vi "NI Selection.vi"(7 "error in (no error)":errorcluster) -> (0 "NI 2":tag, 1 "NI 1":tag, 2 "Ok/Cancel":enum16{"Ok", "Cancel"}(ring), 3 "error out":errorcluster)   [LabVIEW 2017]
uses:
  <resource>/objmgr/daqmx.rc
panel:
  in  "NI2":tag
  in  "NI1":tag
  in  "Cancel Button":bool
  in  "OK Button":bool
  # "PLease Choose Correct NI Serial Number"
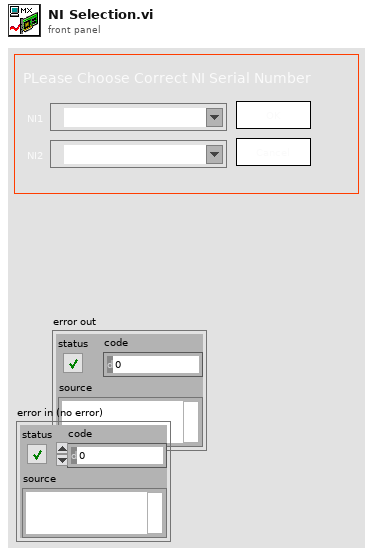
[diagram p1: front panel]
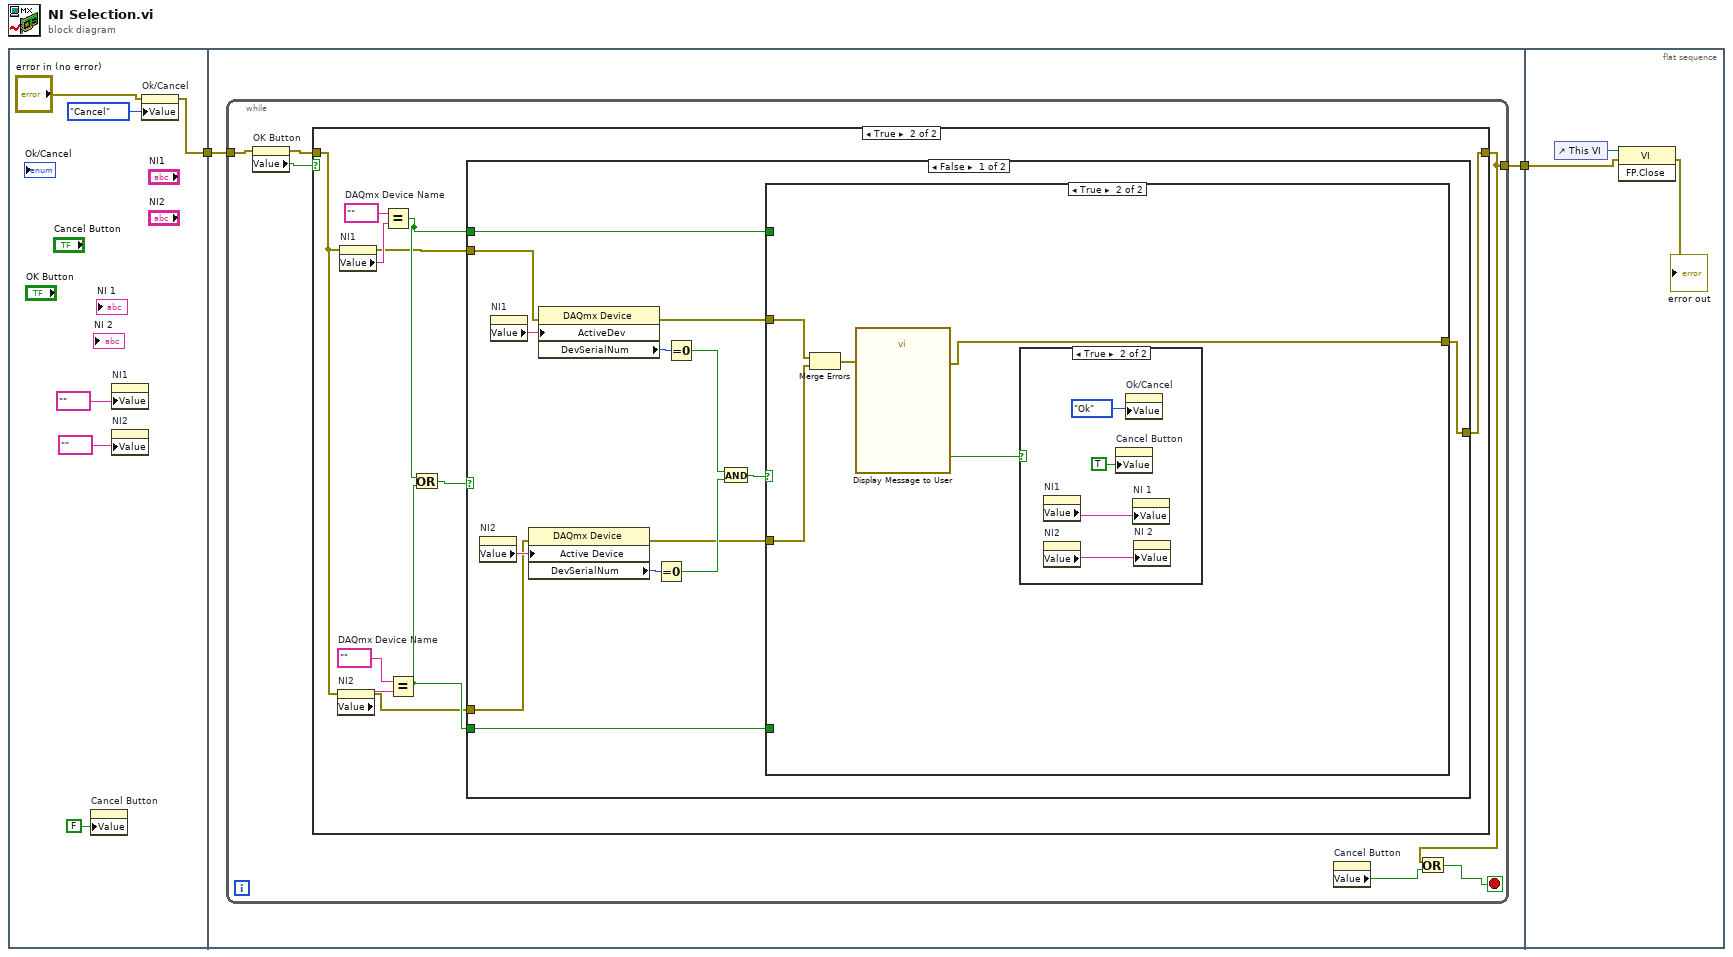
[diagram p0: block diagram]
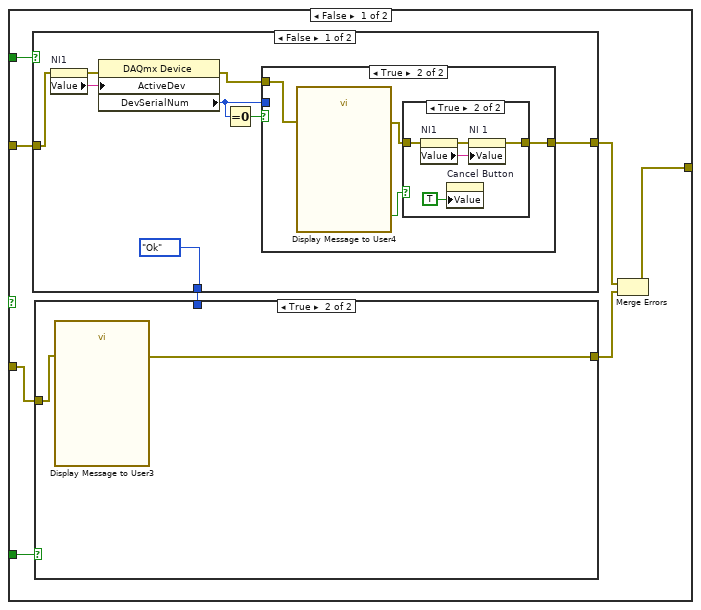
[diagram p3: hidden frame]
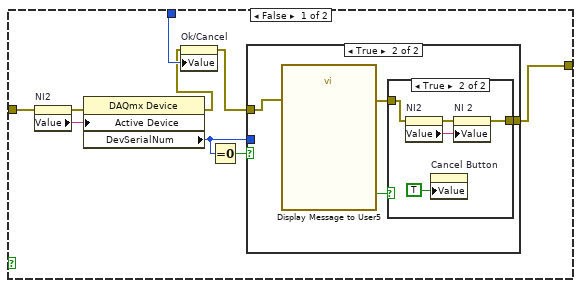
[diagram p4: hidden frame]
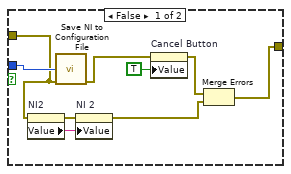
[diagram p5: hidden frame]
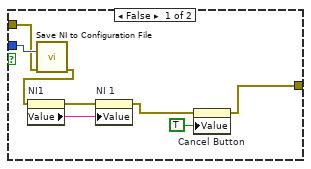
[diagram p7: hidden frame]
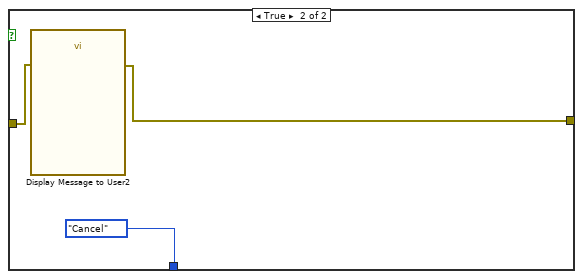
[diagram p9: hidden frame]
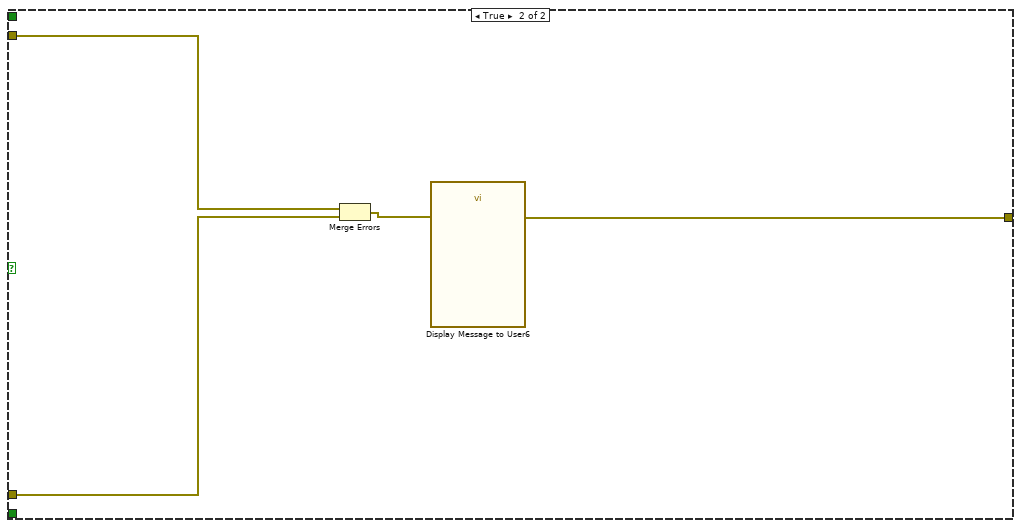
[diagram p11: hidden frame]
diagram:
  n1 = flat-sequence {
    tunnel: [w4] -> w2
    tunnel: w2 -> [w10]
    tunnel: [w9] -> w1
    tunnel: w1 -> [w124]
    frame #0 {
      n2 = property on="Cancel Button" class="Bool (strict)"("Value"=FALSE ("Cancel Button")) -> ()  [unwired: 2 in, 2 out]
      n3 = property on="NI1" class="DAQmxName"("Value"=tag "" ("NI 2")) -> ()  [unwired: 2 in, 2 out]
      n4 = property on="NI2" class="DAQmxName"("Value"=tag "" ("NI 2")) -> ()  [unwired: 2 in, 2 out]
      n5 = property on="Ok/Cancel" class="Enum (strict)"(error in="error in (no error)", "Value"=enum16{"Ok", "Cancel"}."Cancel" ("Ok/Cancel")) -> (error out=w4:errorcluster)  [unwired: 1 in, 1 out]
    }
    frame #1 {
      n6 = while {
        tunnel: w10 -> [w15]
        tunnel: [w11] -> w9
        stop <- w13 stop-if-true
        n7 = property on="OK Button" class="Bool (strict)"(error in=w15) -> (error out=w14:errorcluster, "Value"=w16:bool)  [unwired: 1 in, 1 out]
        n8 = case shown="True" w16 {
          tunnel: [w17 w18] -> w11
          tunnel: w14 -> [w17 w21]
          frame False {
          }
          frame True {
            w25 = tag ""  # DAQmx Device Name
            w28 = tag ""  # DAQmx Device Name
            n9 = property on="NI2" class="DAQmxName"(error in=w21) -> (error out=w19:errorcluster, "Value"=w26:string)  [unwired: 1 in, 1 out]
            n10 = property on="NI1" class="DAQmxName"(error in=w21) -> (error out=w20:errorcluster, "Value"=w27:string)  [unwired: 1 in, 1 out]
            n11 = Equal?(x=w28, y=w27) -> (x = y?=w23:bool)
            n12 = Equal?(x=w25, y=w26) -> (x = y?=w22:bool)
            n13 = Or(x=w23, y=w22) -> (x .or. y?=w24:bool)
            n14 = case shown="False" w24 {
              tunnel: w23 -> [w42 _]
              tunnel: w22 -> [w41 _]
              tunnel: w20 -> [w33 w121]
              tunnel: w19 -> [w32 w120]
              tunnel: [w29 w119] -> w18
              frame False {
                n15 = property on="NI2" class="DAQmxName"() -> ("Value"=w37:string)  [unwired: 2 in, 2 out]
                n16 = property on="NI1" class="DAQmxName"() -> ("Value"=w39:string)  [unwired: 2 in, 2 out]
                n17 = property class="DAQmx Device"(error in=w32, "Active Device"=w37) -> (error out=w30:errorcluster, "DevSerialNum"=w38:u32)  [unwired: 1 in, 1 out]
                n18 = property class="DAQmx Device"(error in=w33, "ActiveDev"=w39) -> (error out=w31:errorcluster, "DevSerialNum"=w40:u32)  [unwired: 1 in, 1 out]
                n19 = Equal To 0?(x=w38) -> (x = 0?=w35:bool)
                n20 = Equal To 0?(x=w40) -> (x = 0?=w36:bool)
                n21 = And(x=w36, y=w35) -> (x .and. y?=w34:bool)
                n22 = case shown="True" w34 {
                  tunnel: w42 -> [w50 _]
                  tunnel: w41 -> [w49 _]
                  tunnel: w31 -> [w47 w113]
                  tunnel: w30 -> [w46 w112]
                  tunnel: [w43 w110] -> w29
                  frame False {
                    n23 = case shown="False" w50 {
                      tunnel: [enum16{"Ok", "Cancel"}."Ok" ("Ok/Cancel") enum16{"Ok", "Cancel"}."Cancel" ("Ok/Cancel")] -> w48
                      tunnel: w47 -> [w83 w107]
                      tunnel: [w81 w108] -> w45
                      frame False {
                        n24 = property on="NI1" class="DAQmxName"(error in=w83) -> (error out=w84:errorcluster, "Value"=w88:string)  [unwired: 1 in, 1 out]
                        n25 = property class="DAQmx Device"(error in=w84, "ActiveDev"=w88) -> (error out=w82:errorcluster, "DevSerialNum"=w86:u32)  [unwired: 1 in, 1 out]
                        n26 = Equal To 0?(x=w86) -> (x = 0?=w87:bool)
                        n27 = case shown="True" w87 {
                          tunnel: w86 -> [w93 _]
                          tunnel: w82 -> [w92 w99]
                          tunnel: [w89 w97] -> w81
                          frame False {
                            n28 = call "Save NI to Configuration File.vi"("NI1"=w93, "error in"=w92) -> ("error out"=w91:errorcluster)  [unwired: 13 in]
                            n29 = property on="NI1" class="DAQmxName"(error in=w91) -> (error out=w96:errorcluster, "Value"=w95:string)  [unwired: 1 in, 1 out]
                            n30 = property on="NI 1" class="DAQmxName"(error in=w96, "Value"=w95) -> (error out=w90:errorcluster)  [unwired: 1 in, 1 out]
                            n31 = property on="Cancel Button" class="Bool (strict)"(error in=w90, "Value"=TRUE ("Cancel Button")) -> (error out=w89:errorcluster)  [unwired: 1 in, 1 out]
                          }
                          frame True {
                            n32 = call "Display Message to User4"("error in (no error)"=w99) -> ("error out"=w98:errorcluster, "OK"=w100:bool)  [unwired: 9 in]
                            n33 = case shown="True" w100 {
                              tunnel: w98 -> [w101 w103]
                              tunnel: [w101 w102] -> w97
                              frame False {
                              }
                              frame True {
                                n34 = property on="NI1" class="DAQmxName"(error in=w103) -> (error out=w106:errorcluster, "Value"=w105:string)  [unwired: 1 in, 1 out]
                                n35 = property on="Cancel Button" class="Bool (strict)"("Value"=TRUE ("Cancel Button")) -> ()  [unwired: 2 in, 2 out]
                                n36 = property on="NI 1" class="DAQmxName"(error in=w106, "Value"=w105) -> (error out=w102:errorcluster)  [unwired: 1 in, 1 out]
                              }
                            }
                          }
                        }
                      }
                      frame True {
                        n37 = call "Display Message to User2"("error in (no error)"=w107) -> ("error out"=w108:errorcluster)  [unwired: 9 in, 1 out]
                      }
                    }
                    n38 = case shown="True" w49 {
                      tunnel: w48 -> [w56 _]
                      tunnel: w46 -> [w55 w80]
                      tunnel: [w51 w79] -> w44
                      frame False {
                        n39 = property on="NI2" class="DAQmxName"(error in=w55) -> (error out=w54:errorcluster, "Value"=w59:string)  [unwired: 1 in, 1 out]
                        n40 = property class="DAQmx Device"(error in=w54, "Active Device"=w59) -> (error out=w52:errorcluster, "DevSerialNum"=w57:u32)  [unwired: 1 in, 1 out]
                        n41 = property on="Ok/Cancel" class="Enum (strict)"(error in=w52, "Value"=w56) -> (error out=w53:errorcluster)  [unwired: 1 in, 1 out]
                        n42 = Equal To 0?(x=w57) -> (x = 0?=w58:bool)
                        n43 = case shown="True" w58 {
                          tunnel: w57 -> [w65 _]
                          tunnel: w53 -> [w63 w71]
                          tunnel: [w60 w69] -> w51
                          frame False {
                            n44 = property on="NI2" class="DAQmxName"(error in=w63) -> (error out=w68:errorcluster, "Value"=w67:string)  [unwired: 1 in, 1 out]
                            n45 = call "Save NI to Configuration File.vi"("NI2"=w65, "error in"=w63) -> ("error out"=w64:errorcluster)  [unwired: 13 in]
                            n46 = property on="NI 2" class="DAQmxName"(error in=w68, "Value"=w67) -> (error out=w61:errorcluster)  [unwired: 1 in, 1 out]
                            n47 = property on="Cancel Button" class="Bool (strict)"(error in=w64, "Value"=TRUE ("Cancel Button")) -> (error out=w62:errorcluster)  [unwired: 1 in, 1 out]
                            n48 = Merge Errors(w62, w61) -> (w60:errorcluster)
                          }
                          frame True {
                            n49 = call "Display Message to User5"("error in (no error)"=w71) -> ("error out"=w70:errorcluster, "OK"=w72:bool)  [unwired: 9 in]
                            n50 = case shown="True" w72 {
                              tunnel: w70 -> [w73 w75]
                              tunnel: [w73 w74] -> w69
                              frame False {
                              }
                              frame True {
                                n51 = property on="NI2" class="DAQmxName"(error in=w75) -> (error out=w78:errorcluster, "Value"=w77:string)  [unwired: 1 in, 1 out]
                                n52 = property on="Cancel Button" class="Bool (strict)"("Value"=TRUE ("Cancel Button")) -> ()  [unwired: 2 in, 2 out]
                                n53 = property on="NI 2" class="DAQmxName"(error in=w78, "Value"=w77) -> (error out=w74:errorcluster)  [unwired: 1 in, 1 out]
                              }
                            }
                          }
                        }
                      }
                      frame True {
                        n54 = call "Display Message to User3"("error in (no error)"=w80) -> ("error out"=w79:errorcluster)  [unwired: 9 in, 1 out]
                      }
                    }
                    n55 = Merge Errors(w45, w44) -> (w43:errorcluster)
                  }
                  frame True {
                    n56 = Merge Errors(w113, w112) -> (w111:errorcluster)
                    n57 = call "Display Message to User"("error in (no error)"=w111) -> ("error out"=w110:errorcluster, "OK"=w114:bool)  [unwired: 9 in]
                    n58 = case shown="True" w114 {
                      frame False {
                      }
                      frame True {
                        n59 = property on="NI1" class="DAQmxName"() -> ("Value"=w116:string)  [unwired: 2 in, 2 out]
                        n60 = property on="NI2" class="DAQmxName"() -> ("Value"=w115:string)  [unwired: 2 in, 2 out]
                        n61 = property on="Cancel Button" class="Bool (strict)"("Value"=TRUE ("Cancel Button")) -> ()  [unwired: 2 in, 2 out]
                        n62 = property on="Ok/Cancel" class="Enum (strict)"("Value"=enum16{"Ok", "Cancel"}."Ok" ("Ok/Cancel")) -> ()  [unwired: 2 in, 2 out]
                        n63 = property on="NI 1" class="DAQmxName"("Value"=w116) -> ()  [unwired: 2 in, 2 out]
                        n64 = property on="NI 2" class="DAQmxName"("Value"=w115) -> ()  [unwired: 2 in, 2 out]
                      }
                    }
                  }
                }
              }
              frame True {
                n65 = Merge Errors(w121, w120) -> (w122:errorcluster)
                n66 = call "Display Message to User6"("error in (no error)"=w122) -> ("error out"=w119:errorcluster)  [unwired: 9 in, 1 out]
              }
            }
          }
        }
        n67 = property on="Cancel Button" class="Bool (strict)"() -> ("Value"=w12:bool)  [unwired: 2 in, 2 out]
        n68 = Or(x=w11, y=w12) -> (x .or. y?=w13:bool)
      }
    }
    frame #2 {
      n69 = control-ref of="This VI"() -> (w125:refnum<vi>)
      n70 = invoke class="VI" method="FP.Close"(reference=w125, error in=w124) -> (error out=→"error out":errorcluster)  [unwired: 1 in, 2 out]
    }
  }
